vi "Vision Published Globals.vi"() -> ()   [LabVIEW 2015]
panel:
  out "Ball Z":dbl
  out "Ball Y":dbl
  out "Ball X":dbl
  out "Confidence in Ball":dbl
  out "Distance to Goal":dbl
  out "Angle to Goal":dbl
  out "Goal Detected":bool
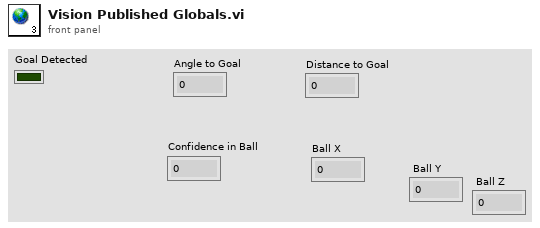
[diagram p1: front panel]
diagram:
